vi "LabVIEW File_ Health Monitoring System.vi"() -> ()   [LabVIEW 2020]
panel:
  out "Battery Status":dbl(graph)
  out "?":bool
  out "power":dbl(graph)
  out "calories":dbl(graph)
  out "speed":dbl(graph)
  in  "PORT NAME":refnum<visa-resource-name>
  in  "Fitness Table":string[][](table)
  out "co2":dbl(graph)
  out "Heart rate BPM":dbl(graph)
  out "CO2 Level":dbl(slide) scale=0.0..1000.0
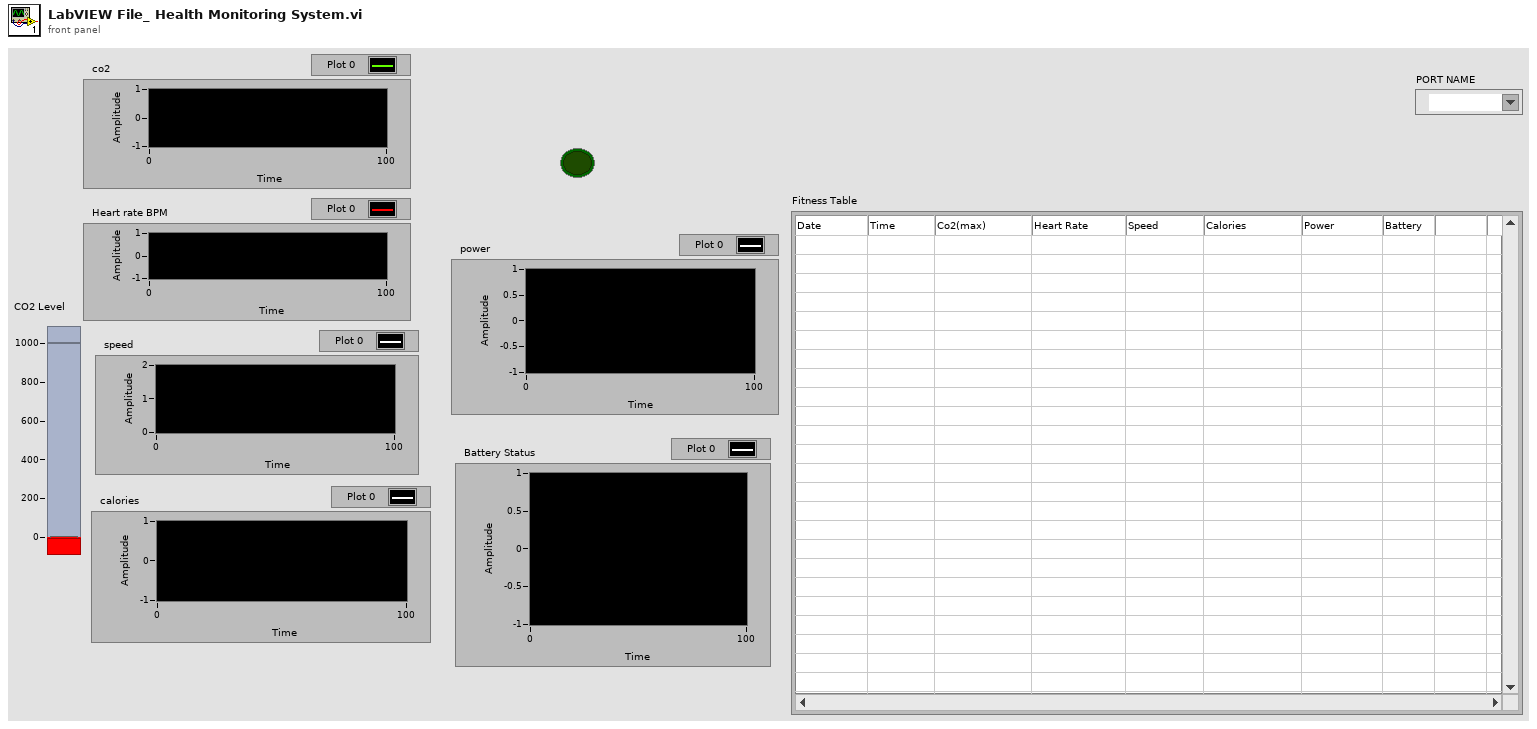
[diagram p1: front panel]
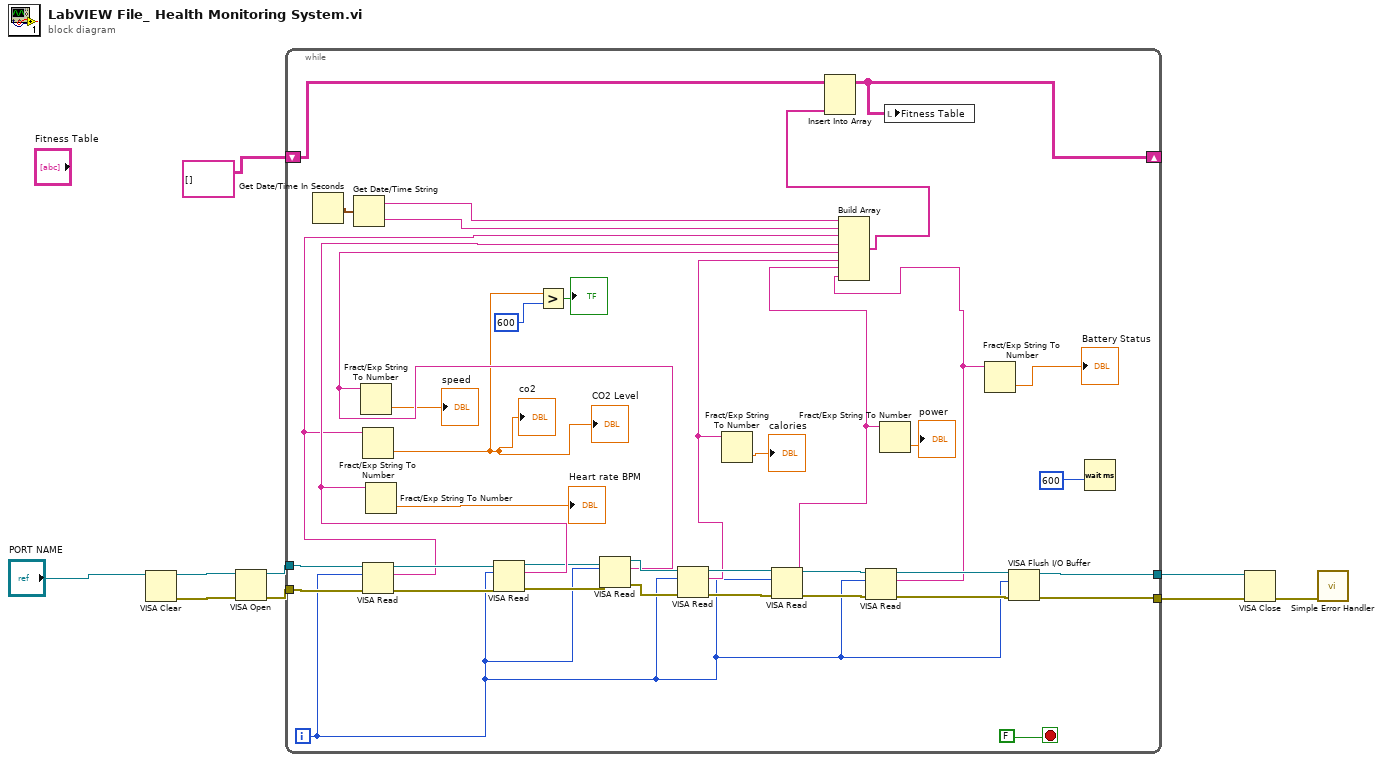
[diagram p0: block diagram]
diagram:
  n1 = VISA Clear(VISA resource name="PORT NAME") -> (VISA resource name out=w8:refnum<visa-resource-name>, error out=w9:errorcluster)  [unwired: 1 in]
  n2 = VISA Open(error in (no error)=w9, VISA resource name=w8) -> (VISA resource name=w7:refnum<visa-resource-name>, error out=w6:errorcluster)  [unwired: 3 in]
  n3 = while {
    tunnel: w7 -> [w48]
    tunnel: w6 -> [w47]
    tunnel: [w37] -> w5
    tunnel: [w30] -> w4
    shift-right: [w21] -> _
    shift-left: string[][] [] -> [w43]
    i -> [w12]
    stop <- FALSE stop-if-true
    n4 = Get Date/Time In Seconds() -> (seconds since 1Jan1904=w42:timestamp)
    n5 = Get Date/Time String(seconds (now)=w42) -> (date string=w41:string, time string=w40:string)  [unwired: 2 in]
    n6 = VISA Read(VISA resource name=w48, byte count=w12, error in (no error)=w47) -> (VISA resource name out=w46:refnum<visa-resource-name>, read buffer=w18:string, error out=w45:errorcluster)  [unwired: 1 out]
    n7 = Fract/Exp String To Number(string=w18) -> (number=w17:dbl)  [unwired: 3 in, 1 out]
    "CO2 Level" <- w17
    "co2" <- w17
    n8 = VISA Read(VISA resource name=w46, byte count=w12, error in (no error)=w45) -> (VISA resource name out=w36:refnum<visa-resource-name>, read buffer=w39:string, error out=w35:errorcluster)  [unwired: 1 out]
    n9 = Fract/Exp String To Number(string=w39) -> (number=→"Heart rate BPM":dbl)  [unwired: 3 in, 1 out]
    n10 = Greater?(x=w17, y=600) -> (0:→"?":bool)
    n11 = VISA Read(VISA resource name=w36, byte count=w12, error in (no error)=w35) -> (VISA resource name out=w34:refnum<visa-resource-name>, read buffer=w28:string, error out=w32:errorcluster)  [unwired: 1 out]
    n12 = Fract/Exp String To Number(string=w28) -> (number=→"speed":dbl)  [unwired: 3 in, 1 out]
    n13 = VISA Read(VISA resource name=w34, byte count=w12, error in (no error)=w32) -> (VISA resource name out=w33:refnum<visa-resource-name>, read buffer=w26:string, error out=w31:errorcluster)  [unwired: 1 out]
    n14 = Fract/Exp String To Number(string=w26) -> (number=→"calories":dbl)  [unwired: 3 in, 1 out]
    n15 = VISA Read(VISA resource name=w33, byte count=w12, error in (no error)=w31) -> (VISA resource name out=w16:refnum<visa-resource-name>, read buffer=w24:string, error out=w15:errorcluster)  [unwired: 1 out]
    n16 = VISA Read(VISA resource name=w16, byte count=w12, error in (no error)=w15) -> (VISA resource name out=w14:refnum<visa-resource-name>, read buffer=w11:string, error out=w13:errorcluster)  [unwired: 1 out]
    n17 = Build Array(w41, w40, w18, w39, w28, w26, w24, w11) -> (w22:string[])
    n18 = Insert Into Array(array=w43, new element=w22) -> (w21:string[][])  [unwired: 2 in]
    n19 = Fract/Exp String To Number(string=w24) -> (number=→"power":dbl)  [unwired: 3 in, 1 out]
    n20 = local write "Fitness Table"(w21) -> ()
    n21 = Fract/Exp String To Number(string=w11) -> (number=→"Battery Status":dbl)  [unwired: 3 in, 1 out]
    n22 = VISA Flush I/O Buffer(VISA resource name=w14, mask (16)=w12, error in (no error)=w13) -> (VISA resource name out=w37:refnum<visa-resource-name>, error out=w30:errorcluster)
    n23 = Wait (ms)(milliseconds to wait=u32 600 ("millisecond timer value")) -> ()  [unwired: 1 out]
  }
  n24 = VISA Close(VISA resource name=w5, error in (no error)=w4) -> (error out=w1:errorcluster)
  n25 = call <vilib>:"Simple Error Handler.vi"("error in (no error)"=w1) -> ()  [unwired: 4 in, 5 out]
